vi "Put - NT.vi"(7 "PV name":string, 8 "error in (no error)":errorcluster, 9 "timeout":dbl[unit]=1.0, 10 "value in":refnum<class "NT Base.lvclass">, 11 "Client in":refnum<class "Client.lvclass">) -> (0 "error out":errorcluster, 1 "timed out?":bool, 2 "value out":refnum<class "NT Base.lvclass">, 3 "Client out":refnum<class "Client.lvclass">)   [LabVIEW 2020, in "PV Access.lvlib" / "PVA Client.lvlib" / "Client.lvclass"]
uses:
  Client.lvclass
  PV Data/NT Base/NT Base.lvclass
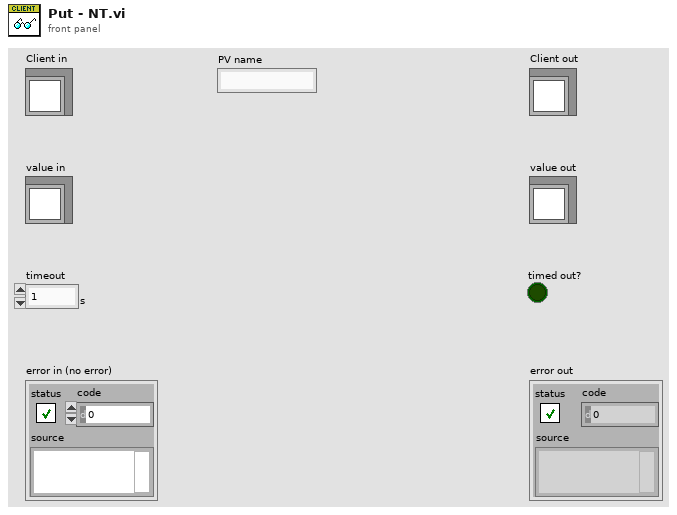
[diagram p1: front panel]
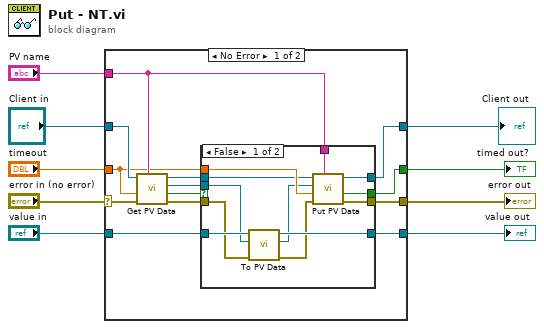
[diagram p0: block diagram]
diagram:
  n1 = case shown="No Error" "error in (no error)" {
    selector: "error in (no error)" -> [w22 w41]
    tunnel: [w16 w41] -> w8
    tunnel: [w10 w40] -> w6
    tunnel: "Client in" -> [w21 w40]
    tunnel: "value in" -> [w20 w39]
    tunnel: [w18 w39] -> w4
    tunnel: "timeout" -> [w14 _]
    tunnel: "PV name" -> [w15 _]
    tunnel: [w13 _] -> w1
    frame No Error {
      n2 = call "Get PV Data.vi"("PV name"=w15, "error in"=w22, "timeout"=w14, "Client in"=w21) -> ("error out"=w19:errorcluster, "timed out?"=w12:bool, "PV Data out"=w17:refnum<class "PV Data.lvclass">, "Client out"=w11:refnum<class "Client.lvclass">)  [unwired: 4 in]
      n3 = case shown="False" w12 {
        selector: w12 -> [_ w35]
        tunnel: w20 -> [w34 w38]
        tunnel: w19 -> [w33 w37]
        tunnel: [w32 w38] -> w18
        tunnel: w17 -> [w31 _]
        tunnel: [w30 w37] -> w16
        tunnel: w15 -> [w28 _]
        tunnel: w14 -> [w27 _]
        tunnel: [w26 w35] -> w13
        tunnel: w11 -> [w25 w36]
        tunnel: [w23 w36] -> w10
        frame False {
          n4 = call-dynamic "To PV Data.vi"("error in (no error)"=w33, "PV Data in"=w31, "Base in"=w34) -> ("error out"=w29:errorcluster, "PV Data out"=w24:refnum<class "PV Data.lvclass">, "Base out"=w32:refnum<class "NT Base.lvclass">)  [unwired: 6 in]
          n5 = call "Put PV Data.vi"("PV name"=w28, "error in"=w29, "timeout"=w27, "PV Data in"=w24, "Client in"=w25) -> ("error out"=w30:errorcluster, "timed out?"=w26:bool, "Client out"=w23:refnum<class "Client.lvclass">)  [unwired: 4 in]
        }
        frame True {
        }
      }
    }
    frame Error {
    }
  }
  "error out" <- w8
  "Client out" <- w6
  "value out" <- w4
  "timed out?" <- w1
